vi "Bookmarks.vi"(8 "Error In":errorcluster, 10 "Reset BM Cache?":bool, 11 "App Info":T1) -> (0 "Error Out":errorcluster, 2 "Possible Undisplayed Bookmarks":bool, 3 "Bookmarks":T2[](array[typedef]))   [LabVIEW 2018, in "Bookmark Manager.lvlib"]
uses:
  Bookmark Manager.lvlib
  Controls/BMark_Bookmark Data.ctl
  Controls/BMark_VI_Identifier.ctl
  <vilib>/addons/analyzer/_analyzerctrls.llb/VIAnCtl Analysis App Info.ctl
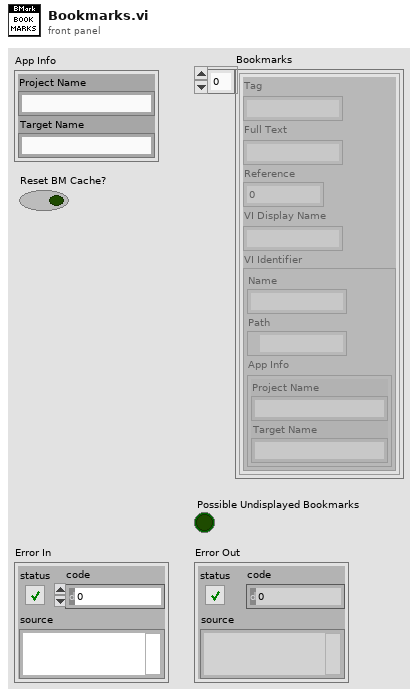
[diagram p1: front panel]
types:
  T1 = typedef "VIAnCtl Analysis App Info.ctl" = cluster{"Project Name":string, "Target Name":string}
  T2 = typedef "Bookmark Manager.lvlib/BMark_Bookmark Data.ctl" = cluster{"Tag":string, "Full Text":string, "Reference":i32, "VI Display Name":string, "VI Identifier":T3}
  T3 = typedef "Bookmark Manager.lvlib/BMark_VI_Identifier.ctl" = cluster{"Name":string, "Path":path, "App Info":T1}
  T4 = typedef "LVBookmarkInfoTypeDef.ctl" = cluster{"Bookmark ID":u32, "Bookmark Tag":string, "Label Text":string}[]
  T5 = typedef "Bookmark Manager.lvlib/BMark_Array of Bookmarks.ctl" = T6[]
  T6 = typedef "Bookmark Manager.lvlib/BMark_Bookmark Cluster.ctl" = cluster{"Reference":i32, "Bookmark":string, "Label Text":string, "VI Identifier":T3}
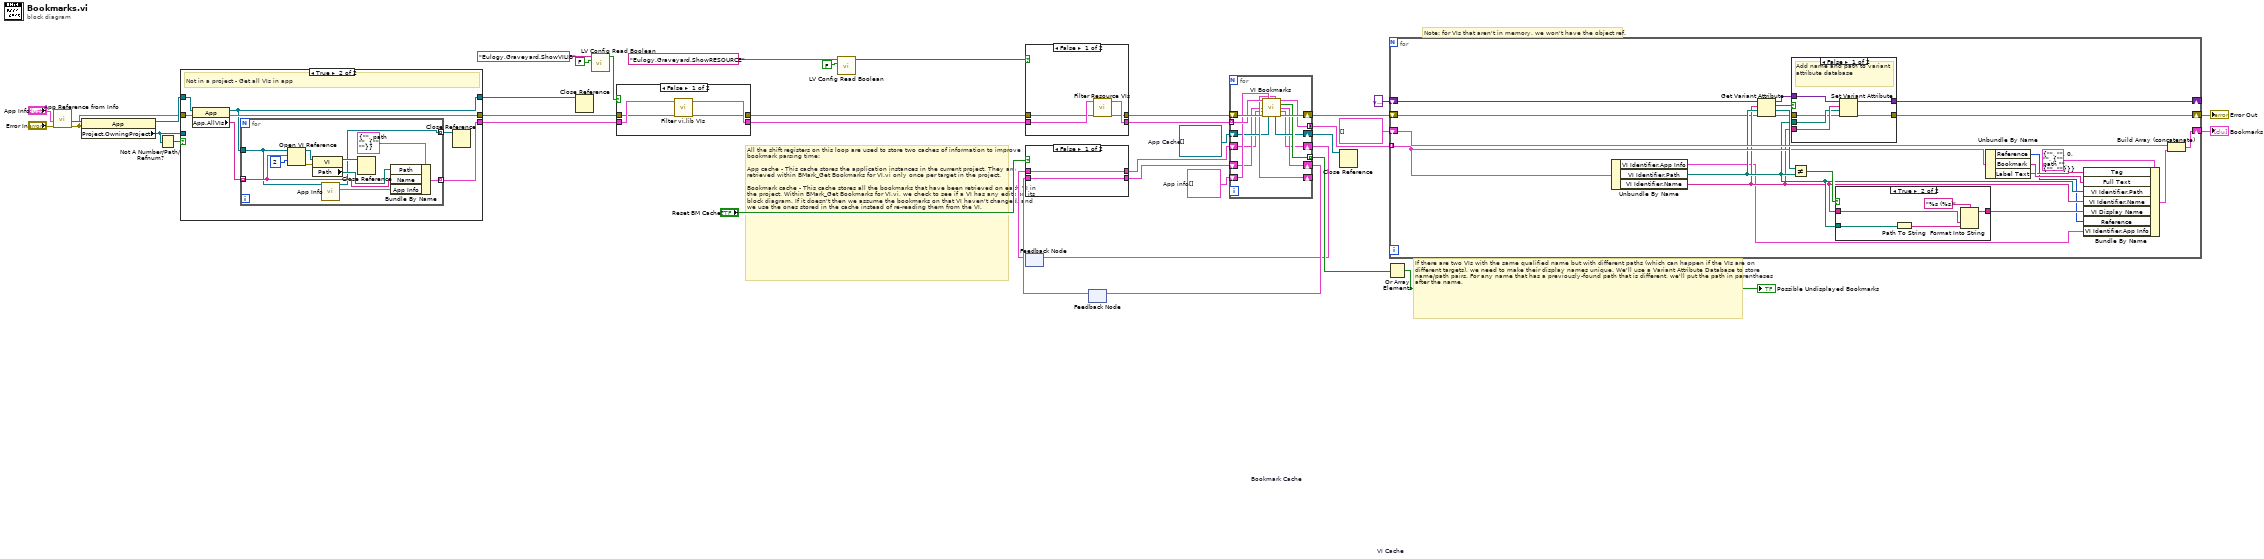
[diagram p0: block diagram]
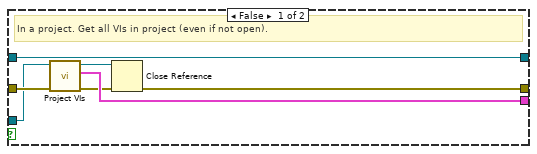
[diagram p5: hidden frame]
diagram:
  w11 = refnum<vi>[] []  # App Cache
  w12 = T1[] []  # App info
  # "All the shift registers on this loop are used to store two caches of information to improve bookmark parsing time:\n\nApp cache - This cache stores the application instances in the current project. They are retrieved within BMark_Get Bookmarks for VI.vi only once per target in the project.\n\nBookmark cache - This cache stores all the bookmarks that have been retrieved on each VI in the project. Within BMark_Get Bookmarks for VI.vi, we check to see if a VI has any edits on its block diagram. If it doesn't then we assume the bookmarks on that VI haven't changed, and we use the ones stored in the cache instead of re-reading them from the VI."
  # "Note: for VIs that aren't in memory, we won't have the object ref."
  # "If there are two VIs with the same qualified name but with different paths (which can happen if the VIs are on different targets), we need to make their display names unique. We'll use a Variant Attribute Database to store name/path pairs. For any name that has a previously-found path that is different, we'll put the path in parentheses after the name."
  n1 = call "App Reference from Info.vi"("Error In"="Error In", "Analysis App Info"="App Info") -> ("Error Out"=w23:errorcluster, "Analysis App Ref"=w25:refnum<vi>)  [unwired: 8 in]
  n2 = property class="App"(reference=w25, error in=w23) -> (reference out=w36:refnum<vi>, "Project.OwningProject"=w35:refnum<vi>)  [unwired: 1 out]
  n3 = Not A Number/Path/Refnum?(number/path/refnum=w35) -> (NaN/Path/Refnum?=w37:bool)
  n4 = case shown="True" w37 {
    tunnel: w36 -> [w43 w52]
    tunnel: w35 -> [w41 _]
    tunnel: [w39 w48] -> w16
    tunnel: w23 -> [w45 w51]
    tunnel: [w44 w49] -> w15
    tunnel: [w43 w47] -> w22
    frame False {
      # "In a project. Get all VIs in project (even if not open)."
      n5 = call "Project VIs.vi"("Error In"=w45, "Project In"=w41) -> ("Error Out"=w42:errorcluster, "VIs"=w44:T3[], "Project Out"=w40:refnum<vi>)  [unwired: 7 in]
      n6 = Close Reference(reference=w40, error in (no error)=w42) -> (error out=w39:errorcluster)
    }
    frame True {
      # "Not in a project - Get all VIs in app"
      n7 = property class="App"(reference=w52, error in=w51) -> (reference out=w47:refnum<vi>, error out=w48:errorcluster, "App.AllVIs"=w50:string[])
      n8 = for {
        tunnel: w50 -> [w58] mode=indexing
        tunnel: [w62] -> w49 mode=indexing
        tunnel: w47 -> [w57]
        tunnel: [w54] -> w46 mode=indexing
        n9 = Open VI Reference(application reference (local)=w57, vi path=w58, options=2) -> (vi reference=w61:refnum<vi>, error out=w60:errorcluster)  [unwired: 3 in]
        n10 = property class="VI"(reference=w61, error in=w60) -> (reference out=w56:refnum<vi>, "Path"=w59:path)  [unwired: 1 out]
        n11 = call "App Info.vi"("App Refnum"=w57) -> ("App Info"=w53:T1, "App Refnum for Opening VI"=w54:refnum<vi>)  [unwired: 8 in, 1 out]
        n12 = Close Reference(reference=w56) -> ()  [unwired: 1 in, 1 out]
        n13 = Bundle By Name(cluster=T3 {"Name"="", "Path"=path "", "App Info"={"Project Name"="", "Target Name"=""}} ("Cluster"), "Path"=w59, "Name"=w58, "App Info"=w53) -> (w62:T3)
      }
      n14 = Close Reference(reference=w46) -> ()  [unwired: 1 in, 1 out]
    }
  }
  n15 = Close Reference(reference=w22) -> ()  [unwired: 1 in, 1 out]
  n16 = call <resource>:"LV Config Read Boolean.vi"("default value"=FALSE, "key"="Eulogy.Graveyard.ShowVILIB") -> ("value"=w30:bool)  [unwired: 3 in, 2 out]
  n17 = case shown="False" w30 {
    tunnel: w16 -> [w65 w69]
    tunnel: [w64 w69] -> w20
    tunnel: w15 -> [w67 w68]
    tunnel: [w66 w68] -> w17
    frame False {
      n18 = call "Filter vi.lib VIs.vi"("Error In"=w65, "VIs In"=w67) -> ("Error Out"=w64:errorcluster, "VIs Out"=w66:T3[])  [unwired: 8 in]
    }
    frame True {
    }
  }
  n19 = call <resource>:"LV Config Read Boolean.vi"("default value"=FALSE, "key"="Eulogy.Graveyard.ShowRESOURCE") -> ("value"=w13:bool)  [unwired: 3 in, 2 out]
  n20 = case shown="False" w13 {
    tunnel: w20 -> [w70 w75]
    tunnel: [w71 w75] -> w19
    tunnel: w17 -> [w73 w74]
    tunnel: [w72 w74] -> w18
    frame False {
      n21 = call "Filter Resource VIs.vi"("Error In"=w70, "VIs In"=w73) -> ("Error Out"=w71:errorcluster, "VIs Out"=w72:T3[])  [unwired: 8 in]
    }
    frame True {
    }
  }
  n22 = feedback #1 "Bookmark Cache"() -> (w5:cluster{"BookmarkInfo":T4}[])  [unwired: 1 in]
  n23 = feedback #2 "VI Cache"() -> (w7:T3[])  [unwired: 1 in]
  n24 = case shown="False" "Reset BM Cache?" {
    tunnel: [w77 _] -> w8
    tunnel: w7 -> [w77 _]
    tunnel: [w76 _] -> w6
    tunnel: w5 -> [w76 _]
    frame False {
    }
    frame True {
    }
  }
  n25 = for {
    shift-right: [w89] -> w33
    shift-left: w19 -> [w90]
    tunnel: [w88] -> w34 mode=concatenating
    tunnel: w18 -> [w87] mode=indexing
    tunnel: [w86] -> w28 mode=indexing
    shift-right: [w84] -> _
    shift-left: w12 -> [w85]
    shift-right: [w82] -> w10
    shift-left: w11 -> [w83]
    shift-right: [w81] -> w9
    shift-left: w8 -> [w79]
    shift-right: [w80] -> w3
    shift-left: w6 -> [w78]
    n26 = call "VI Bookmarks.vi"("VI"=w87, "App Infos In"=w85, "VI Cache In"=w79, "Bookmark Cache In"=w78, "Error In"=w90, "App Cache In"=w83) -> ("App Infos Out"=w84:T1[], "Bookmarks"=w88:T5, "Possible Undisplayed Bookmarks"=w86:bool, "VI Cache Out"=w81:T3[], "Bookmark Cache Out"=w80:cluster{"BookmarkInfo":T4}[], "App Cache Out"=w82:refnum<vi>[], "Error Out"=w89:errorcluster)  [unwired: 3 in]
  }
  n27 = feedback-in #1(w3) -> ()
  n28 = feedback-in #2(w9) -> ()
  n29 = Close Reference(reference=w10) -> ()  [unwired: 1 in, 1 out]
  n30 = Or Array Elements(Boolean array=w28) -> (logical OR=→"Possible Undisplayed Bookmarks":bool)
  n31 = for {
    shift-right: [w110] -> w38
    shift-left: T2[] [] -> [w111]
    tunnel: w34 -> [w96] mode=indexing
    shift-right: [w97] -> w32
    shift-left: w33 -> [w93]
    shift-right: [w105] -> _
    shift-left: variant -> [w104]
    n32 = Unbundle By Name(w96) -> ("VI Identifier.App Info"=w91:T1, "VI Identifier.Path"=w95:path, "VI Identifier.Name"=w94:string)
    n33 = Get Variant Attribute(Variant=w104, name=w94, default value (empty Variant)=w95, error in=w93) -> (duplicate Variant=w100:variant, found=w99:bool, value=w103:path, error out=w98:errorcluster)
    n34 = case shown="False" w99 {
      tunnel: [w117 w119] -> w105
      tunnel: w100 -> [w116 w119]
      tunnel: w94 -> [w115 _]
      tunnel: w95 -> [w114 _]
      tunnel: w98 -> [w113 w118]
      tunnel: [w112 w118] -> w97
      frame False {
        # "Add name and path to variant attribute database"
        n35 = Set Variant Attribute(Variant=w116, name=w115, value=w114, error in=w113) -> (Variant out=w117:variant, error out=w112:errorcluster)  [unwired: 1 out]
      }
      frame True {
      }
    }
    n36 = Not Equal?(x=w103, y=w95) -> (x != y?=w101:bool)
    n37 = case shown="True" w101 {
      tunnel: w95 -> [_ w123]
      tunnel: w94 -> [w120 w122]
      tunnel: [w120 w121] -> w102
      frame False {
      }
      frame True {
        n38 = Path To String(path=w123) -> (string=w124:string)
        n39 = Format Into String(format string="%s (%s)", w122, w124) -> (resulting string=w121:string)  [unwired: 2 in, 1 out]
      }
    }
    n40 = Unbundle By Name(w96) -> ("Reference"=w92:i32, "Bookmark"=w106:string, "Label Text"=w107:string)
    n41 = Bundle By Name(cluster=T2 {"Tag"="", "Full Text"="", "Reference"=0, "VI Display Name"="", "VI Identifier"={"Name"="", "Path"=path "", "App Info"={"Project Name"="", "Target Name"=""}}} ("bookmark item"), "Tag"=w106, "Full Text"=w107, "VI Identifier.Path"=w95, "VI Identifier.Name"=w94, "VI Display Name"=w102, "Reference"=w92, "VI Identifier.App Info"=w91) -> (w108:T2)
    n42 = Build Array (concatenate)(w111, w108) -> (w110:T2[])
  }
  "Bookmarks" <- w38
  "Error Out" <- w32
